vi "Scale Image.vi"(8 "error in (no error)":errorcluster, 10 "Selected Data":T1, 11 "Picture in":refnum<vi>) -> (0 "error out":errorcluster)   [LabVIEW 2019]
uses:
  <vilib>/picture/picture.llb/imagedata.ctl
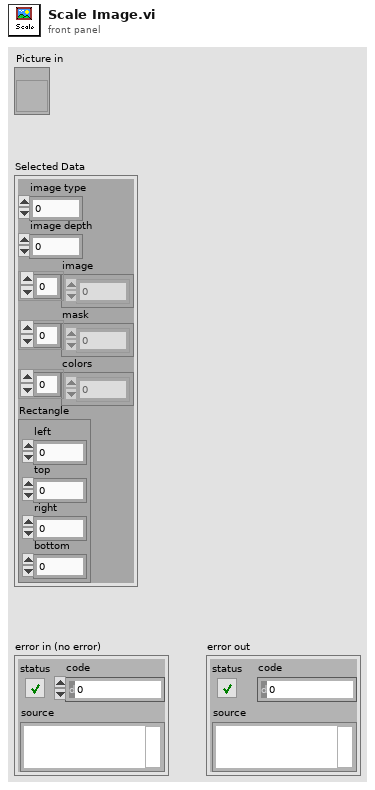
[diagram p1: front panel]
types:
  T1 = typedef "imagedata.ctl" = cluster{"image type":i32, "image depth":i32, "image":u8[], "mask":u8[], "colors":u32[], "Rectangle":cluster{"left":i16, "top":i16, "right":i16, "bottom":i16}}
  T2 = typedef "LVBoundsTypeDef.ctl" = cluster{"Width":u32, "Height":u32}
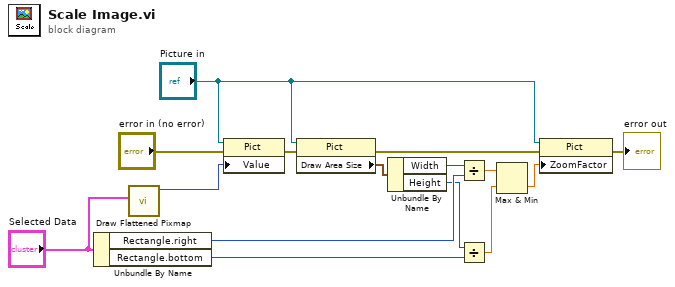
[diagram p0: block diagram]
diagram:
  n1 = Unbundle By Name("Selected Data") -> ("Rectangle.right"=w9:i16, "Rectangle.bottom"=w7:i16)
  n2 = call <vilib>:"Draw Flattened Pixmap.vi"("image data"="Selected Data") -> ("new picture"=w15:picture)  [unwired: 8 in]
  n3 = property on="Property Node" class="Pict"(reference="Picture in", error in="error in (no error)", "Value"=w15) -> (error out=w4:errorcluster)  [unwired: 1 out]
  n4 = property on="Property Node" class="Pict"(reference="Picture in", error in=w4) -> (error out=w3:errorcluster, "Draw Area Size"=w13:T2)  [unwired: 1 out]
  n5 = Unbundle By Name(w13) -> ("Width"=w10:u32, "Height"=w8:u32)
  n6 = Divide(x=w10, y=w9) -> (x/y=w12:dbl)
  n7 = Divide(x=w8, y=w7) -> (x/y=w11:dbl)
  n8 = Max & Min(x=w12, y=w11) -> (min(x,y)=w6:dbl)  [unwired: 1 out]
  n9 = property on="Property Node" class="Pict"(reference="Picture in", error in=w3, "ZoomFactor"=w6) -> (error out=→"error out":errorcluster)  [unwired: 1 out]
